vi "DummyValues.vi"(8 "error in (no error)":errorcluster) -> (0 "error out":errorcluster, 3 "CalibReport out":refnum<class "CalibReport.lvclass">)   [LabVIEW 2024, in "CalibReport.lvclass"]
uses:
  CalibReport.lvclass
  CalibReport.lvclass/CalibReport.ctl
  cReportEntry.ctl
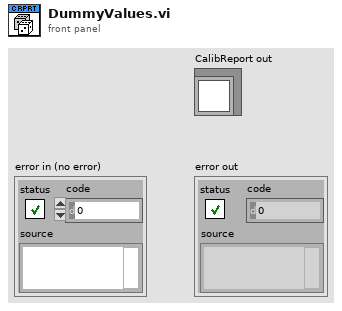
[diagram p1: front panel]
types:
  T1 = typedef "cReportEntry.ctl" = cluster{"Reference [kg]":dbl, "DUT value [kg]":dbl}
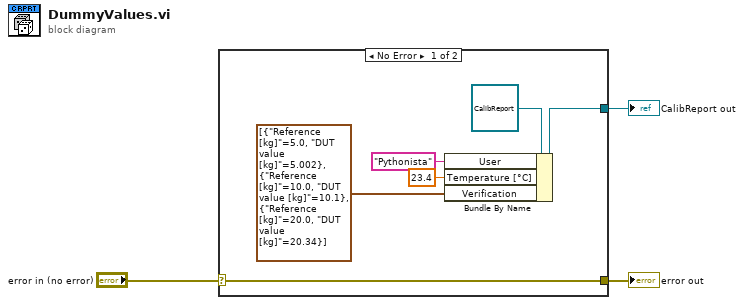
[diagram p0: block diagram]
diagram:
  n1 = case shown="No Error" "error in (no error)" {
    selector: "error in (no error)" -> [w9 w10]
    tunnel: [w9 w10] -> w2
    tunnel: [w8 _] -> w1
    frame No Error {
      n2 = Bundle By Name(cluster=refnum<class "CalibReport.lvclass"> refnum ("CalibReport in"), "User"="Pythonista", "Temperature [°C]"=23.4, "Verification"=T1[] [{"Reference [kg]"=5.0, "DUT value [kg]"=5.002}, {"Reference [kg]"=10.0, "DUT value [kg]"=10.1}, {"Reference [kg]"=20.0, "DUT value [kg]"=20.34}]) -> (w8:refnum<class "CalibReport.lvclass">)
    }
    frame Error {
    }
  }
  "error out" <- w2
  "CalibReport out" <- w1
